vi "Local Assign Point Ramping.vi"(4 "Vac Digital Cmd":i8, 5 "Ramp Time [sec]":dbl=3.0, 6 "L1 to L4 PID Cluster":T1={"L1 PID Gains"={"Kp"=0.005, "Kd"=0.5, "Ki"=0.0005}, "L2 PID Gains"={"Kp"=0.01, "Kd"=1.0, "Ki"=0.0005}, "L3 PID Gains"={"Kp"=0.05, "Kd"=1.0, "Ki"=0.0005}, "L4 PID Gains"={"Kp"=0.1, "Kd"=0.1, "Ki"=0.0005}}, 7 "Offset Home2RCM":dbl[](array[numeric])=[0.0, 0.0, 0.0, 0.0], 8 "Destination Posit Array [mm]":dbl[](array[numeric])=[0.0, 0.0, -3.0, 0.0], 9 "Previous Posit Array":dbl[](array[numeric])=[0.0, 0.0, 0.0, 0.0], 10 "error in":errorcluster, 11 "FPGA VI Reference In":refnum<k20>) -> (1 "Last L1 to L4 Posit":dbl[](array[numeric]), 2 "error out":errorcluster, 3 "FPGA VI Reference Out":refnum<k20>)   [LabVIEW 2016]
uses:
  <vilib>/Analysis/1siggen.llb/Ramp Pattern by Samples.vi
  Subsystems/Global Variables.vi
  <vilib>/Analysis/NI_AALBase.lvlib
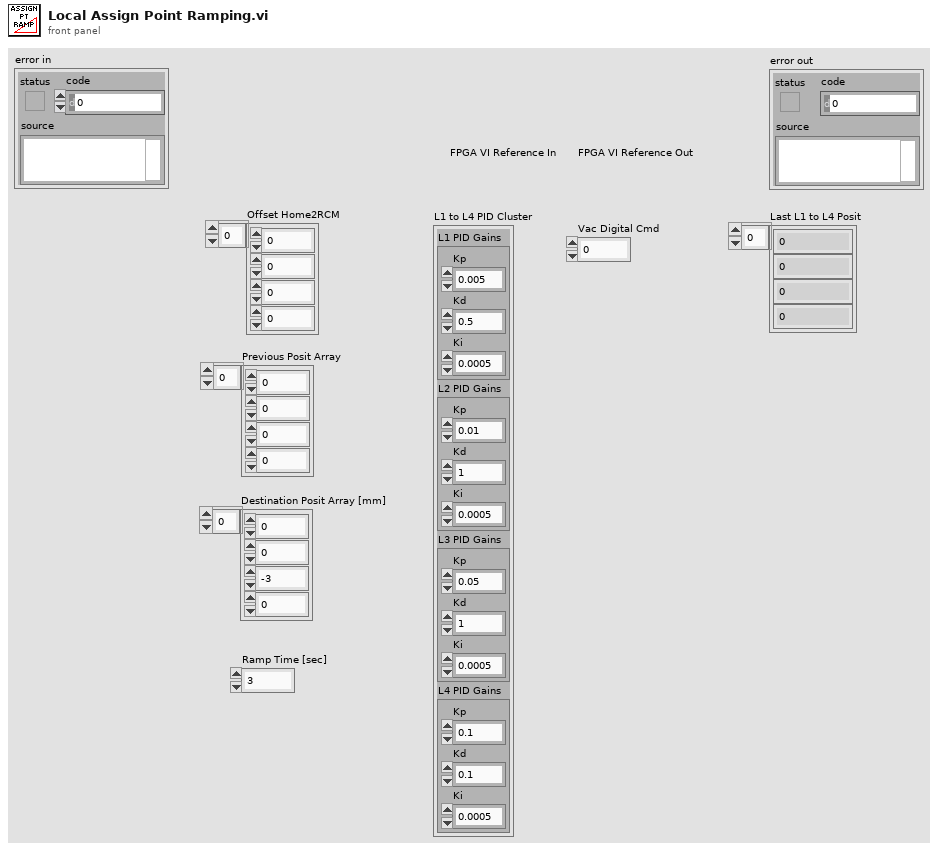
[diagram p1: front panel]
types:
  T1 = cluster{"L1 PID Gains":cluster{"Kp":dbl, "Kd":dbl, "Ki":dbl}, "L2 PID Gains":cluster{"Kp":dbl, "Kd":dbl, "Ki":dbl}, "L3 PID Gains":cluster{"Kp":dbl, "Kd":dbl, "Ki":dbl}, "L4 PID Gains":cluster{"Kp":dbl, "Kd":dbl, "Ki":dbl}}
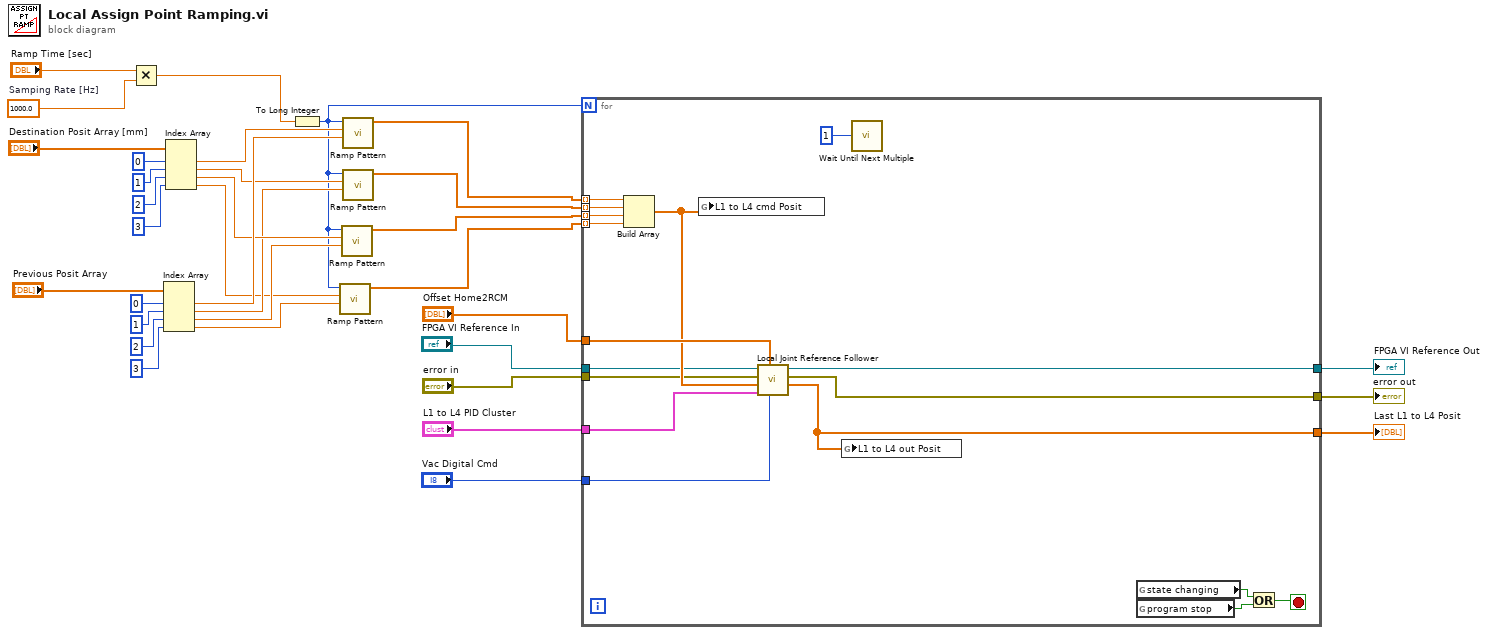
[diagram p0: block diagram]
diagram:
  w23 = 1000.0  # Samping Rate [Hz]
  n1 = Multiply(x="Ramp Time [sec]", y=w23) -> (x*y=w14:dbl)
  n2 = Index Array(array="Previous Posit Array", index #1=0 ("index"), index #2=1 ("index"), index #3=2 ("index"), index #4=3 ("index")) -> (element #1=w22:dbl, element #2=w18:dbl, element #3=w17:dbl, element #4=w16:dbl)
  n3 = Index Array(array="Destination Posit Array [mm]", index #1=0 ("index"), index #2=1 ("index"), index #3=2 ("index"), index #4=3 ("index")) -> (element #1=w21:dbl, element #2=w20:dbl, element #3=w19:dbl, element #4=w15:dbl)
  n4 = To Long Integer(number=w14) -> (32bit integer=w13:i32)
  n5 = call-poly <vilib>:"Ramp Pattern.vi"("start"=w16, "end"=w15, "samples"=w13) -> ("Ramp Pattern"=w9:dbl[])  [unwired: 7 in, 1 out]
  n6 = call-poly <vilib>:"Ramp Pattern.vi"("start"=w17, "end"=w19, "samples"=w13) -> ("Ramp Pattern"=w10:dbl[])  [unwired: 7 in, 1 out]
  n7 = call-poly <vilib>:"Ramp Pattern.vi"("start"=w22, "end"=w21, "samples"=w13) -> ("Ramp Pattern"=w12:dbl[])  [unwired: 7 in, 1 out]
  n8 = call-poly <vilib>:"Ramp Pattern.vi"("start"=w18, "end"=w20, "samples"=w13) -> ("Ramp Pattern"=w11:dbl[])  [unwired: 7 in, 1 out]
  n9 = for {
    N: w13 -> [_]
    tunnel: w12 -> [w51] mode=indexing
    tunnel: w11 -> [w50] mode=indexing
    tunnel: w10 -> [w49] mode=indexing
    tunnel: w9 -> [w48] mode=indexing
    tunnel: [w47] -> w2
    tunnel: [w46] -> w5
    tunnel: "Offset Home2RCM" -> [w45]
    tunnel: "L1 to L4 PID Cluster" -> [w44]
    tunnel: [w42] -> w7
    tunnel: "FPGA VI Reference In" -> [w40]
    tunnel: "error in" -> [w39]
    tunnel: "Vac Digital Cmd" -> [w35]
    stop <- w36 stop-if-true
    n10 = Build Array(w51, w50, w49, w48) -> (w43:dbl[])
    n11 = global write "Global Variables.vi" "L1 to L4 cmd Posit"(w43) -> ()
    n12 = call "Local Joint Reference Follower.vi"("Digital Cmd [0-78]"=w35, "Offset Home2RCM [deg/mm]"=w45, "PID Ctrl Cluster"=w44, "Ref Array [deg/mm]"=w43, "error in"=w39, "FPGA VI Reference In"=w40) -> ("Output Posit Array [deg/mm]"=w42:dbl[], "error out"=w46:errorcluster, "FPGA VI Reference Out"=w47:refnum<k20>)  [unwired: 3 in]
    n13 = global write "Global Variables.vi" "L1 to L4 out Posit"(w42) -> ()
    n14 = call "Wait Until Next Multiple"("Count(mSec)"=u32 1) -> ()  [unwired: 1 out]
    n15 = global read "Global Variables.vi" "state changing"() -> (w38:bool)
    n16 = global read "Global Variables.vi" "program stop"() -> (w37:bool)
    n17 = Or(x=w38, y=w37) -> (x .or. y?=w36:bool)
  }
  "error out" <- w5
  "Last L1 to L4 Posit" <- w7
  "FPGA VI Reference Out" <- w2
